vi "read_plc_datasocket.vi"() -> ()   [LabVIEW 2011]
panel:
  out "LB201_B226_GT402":string
  out "LB201_B226_GP102":string
  out "LB201_B226_GT401":string
  out "LB201_B226_GP101":string
  out "LB201_B226_GT301":string
  out "LB201_B226_U201":string
  out "LB201_B226_GT101":string
  out "KB3_B226_U201":string
  out "KB3_B226_GT401":string
  out "KB3_B226_GP101":string
  out "KB3_B226_GT101":string
  out "VS201_B226_GT301":string
  out "VS201_B226_GP101":string
  out "VS201_B226_GT401":string
  out "VS201_B226_GT101":string
  out "VS201_B226_U201":string
  out "Elapsed Time":dbl
  out "Command":string
  out "Up Time":string
  out "Startup Time":string
  out "Version":string
  out "LB201_B230_SV201":string
  out "LB201_B230_SV401":string
  out "LB201_B230_ST902":string
  out "LB201_B230_ST901":string
  out "LB201_A213_SV201":string
  out "LB201_A213_ST902":string
  out "LB201_A235_SV401":string
  out "LB201_A235_SV201":string
  out "LB201_A235_ST902":string
  out "LB201_A235_ST901":string
  out "LB201_A225_SV401":string
  out "LB201_A225_SV201":string
  out "LB201_A225_ST902":string
  out "LB201_A225_ST901":string
  out "LB201_A213_SV401":string
  out "LB201_A213_ST901":string
  out "LB201_B230_GQ101":string
  out "LB201_B230_GT101":string
  out "LB201_A235_GQ101":string
  out "LB201_A235_GT101":string
  out "LB201_B230_GN501":string
  out "LB201_A235_GN501":string
  out "LB201_A225_GT101":string
  out "LB201_A225_GQ101":string
  out "LB201_A225_GN501":string
  out "LB201_A213_GT101":string
  out "LB201_A213_GQ101":string
  out "LB201_A213_GN501":string
  out "Deque error":errorcluster
  out "DataSocket error":errorcluster
  out "# Sent Data":u64
  # "OPC Server Status"
  # "AI PLCs (Per Room)"
  # "AI PLCs (Common)"
  # "AO PLCs (Per Room)"
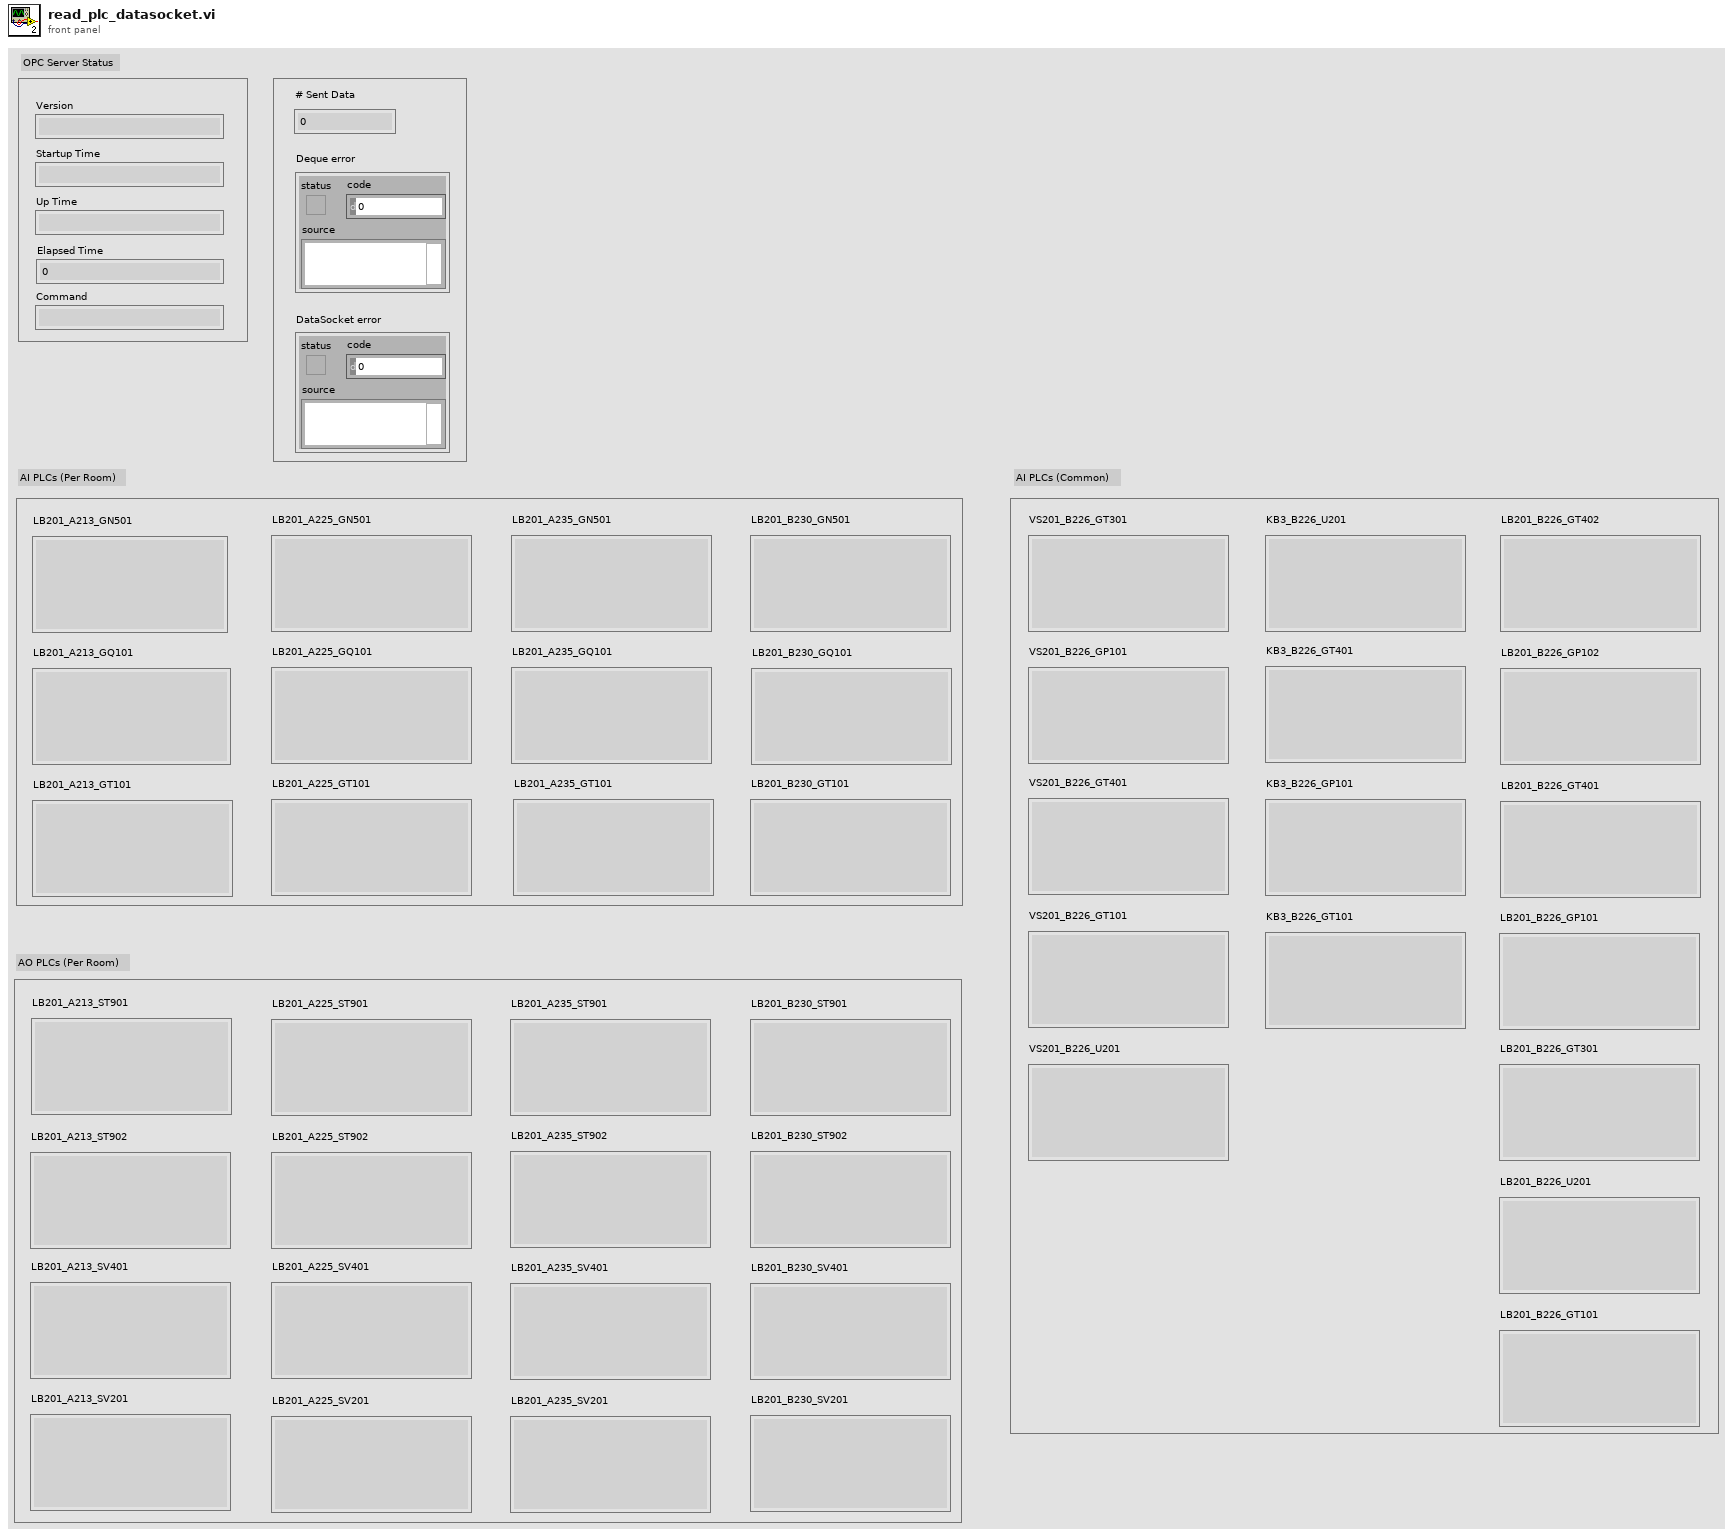
[diagram p1: front panel]
types:
  T1 = enum16{"Read", "Write", "ReadWrite", "BufferedRead", "BufferedReadWrite"}
diagram:
  w3 = string[] ["opc://localhost/Fidelix.FdxOPC/AS_KTH.AI.VS201_B226_GT301_MV.Value", "opc://localhost/Fidelix.FdxOPC/AS_KTH.AI.VS201_B226_GP101_MV.Value", "opc://localhost/Fidelix.FdxOPC/AS_KTH.AI.VS201_B226_GT401_MV.Value", "opc://localhost/Fidelix.FdxOPC/AS_KTH.AI.VS201_B226_GT101_MV.Value", "opc://localhost/Fidelix.FdxOPC/AS_KTH.AI.VS201_B226_U201_SS.Value", "opc://localhost/Fidelix.FdxOPC/AS_KTH.AI.KB3_B226_U201_SS.Value", "opc://localhost/Fidelix.FdxOPC/AS_KTH.AI.KB3_B226_GT401_MV.Value", "opc://localhost/Fidelix.FdxOPC/AS_KTH.AI.KB3_B226_GP101_MV.Value", "opc://localhost/Fidelix.FdxOPC/AS_KTH.AI.KB3_B226_GT101_MV.Value", "opc://localhost/Fidelix.FdxOPC/AS_KTH.AI.LB201_B226_GT402_MV.Value", "opc://localhost/Fidelix.FdxOPC/AS_KTH.AI.LB201_B226_GP102_MV.Value", "opc://localhost/Fidelix.FdxOPC/AS_KTH.AI.LB201_B226_GT401_MV.Value", "opc://localhost/Fidelix.FdxOPC/AS_KTH.AI.LB201_B226_GP101_MV.Value", "opc://localhost/Fidelix.FdxOPC/AS_KTH.AI.LB201_B226_GT301_MV.Value", "opc://localhost/Fidelix.FdxOPC/AS_KTH.AI.LB201_B226_U201_SS.Value", "opc://localhost/Fidelix.FdxOPC/AS_KTH.AI.LB201_B226_GT101_MV.Value"]  # Predefined items
  w32 = string[] ["opc://localhost/Fidelix.FdxOPC/AS_KTH.AI.LB201_A213_ST901_SS.Value", "opc://localhost/Fidelix.FdxOPC/AS_KTH.AI.LB201_A213_ST902_SS.Value", "opc://localhost/Fidelix.FdxOPC/AS_KTH.AI.LB201_A213_SV201_SS.Value", "opc://localhost/Fidelix.FdxOPC/AS_KTH.AI.LB201_A213_SV401_SS.Value", "opc://localhost/Fidelix.FdxOPC/AS_KTH.AI.LB201_A225_ST901_SS.Value", "opc://localhost/Fidelix.FdxOPC/AS_KTH.AI.LB201_A225_ST902_SS.Value", "opc://localhost/Fidelix.FdxOPC/AS_KTH.AI.LB201_A225_SV201_SS.Value", "opc://localhost/Fidelix.FdxOPC/AS_KTH.AI.LB201_A225_SV401_SS.Value", "opc://localhost/Fidelix.FdxOPC/AS_KTH.AI.LB201_A235_ST901_SS.Value", "opc://localhost/Fidelix.FdxOPC/AS_KTH.AI.LB201_A235_ST902_SS.Value", "opc://localhost/Fidelix.FdxOPC/AS_KTH.AI.LB201_A235_SV201_SS.Value", "opc://localhost/Fidelix.FdxOPC/AS_KTH.AI.LB201_A235_SV401_SS.Value", "opc://localhost/Fidelix.FdxOPC/AS_KTH.AI.LB201_B230_ST901_SS.Value", "opc://localhost/Fidelix.FdxOPC/AS_KTH.AI.LB201_B230_ST902_SS.Value", "opc://localhost/Fidelix.FdxOPC/AS_KTH.AI.LB201_B230_SV201_SS.Value", "opc://localhost/Fidelix.FdxOPC/AS_KTH.AI.LB201_B230_SV401_SS.Value"]  # Predefined items
  w37 = string[] ["opc://localhost/Fidelix.FdxOPC/AS_KTH.AI.LB201_A213_GN501_I.Value", "opc://localhost/Fidelix.FdxOPC/AS_KTH.AI.LB201_A213_GQ101_MV.Value", "opc://localhost/Fidelix.FdxOPC/AS_KTH.AI.LB201_A213_GT101_MV.Value", "opc://localhost/Fidelix.FdxOPC/AS_KTH.AI.LB201_A225_GN501_I.Value", "opc://localhost/Fidelix.FdxOPC/AS_KTH.AI.LB201_A225_GQ101_MV.Value", "opc://localhost/Fidelix.FdxOPC/AS_KTH.AI.LB201_A225_GT101_MV.Value", "opc://localhost/Fidelix.FdxOPC/AS_KTH.AI.LB201_A235_GN501_I.Value", "opc://localhost/Fidelix.FdxOPC/AS_KTH.AI.LB201_A235_GQ101_MV.Value", "opc://localhost/Fidelix.FdxOPC/AS_KTH.AI.LB201_A235_GT101_MV.Value", "opc://localhost/Fidelix.FdxOPC/AS_KTH.AI.LB201_B230_GN501_I.Value", "opc://localhost/Fidelix.FdxOPC/AS_KTH.AI.LB201_B230_GQ101_MV.Value", "opc://localhost/Fidelix.FdxOPC/AS_KTH.AI.LB201_B230_GT101_MV.Value"]  # Predefined items
  n1 = for {
    tunnel: w37 -> [w48] mode=indexing
    tunnel: [w47] -> w36 mode=indexing
    tunnel: [w46] -> w35 mode=indexing
    n2 = DataSocket Open(10:T1."Read" ("mode"), 11:w48) -> (0:w46:errorcluster, 3:w47:refnum<k13>)  [unwired: 1 in, 1 out]
  }
  n3 = DataSocket Open(10:T1."Read" ("mode"), 11:"opc://localhost/Fidelix.FdxOPC/ServerStatus.Version" ("URL")) -> (0:w16:errorcluster, 3:w17:refnum<k13>)  [unwired: 1 in, 1 out]
  n4 = DataSocket Open(10:T1."Read" ("mode"), 11:"opc://localhost/Fidelix.FdxOPC/ServerStatus.StartupTime" ("URL")) -> (0:w14:errorcluster, 3:w15:refnum<k13>)  [unwired: 1 in, 1 out]
  n5 = DataSocket Open(10:T1."Read" ("mode"), 11:"opc://localhost/Fidelix.FdxOPC/ServerStatus.UpTime" ("URL")) -> (0:w12:errorcluster, 3:w13:refnum<k13>)  [unwired: 1 in, 1 out]
  n6 = DataSocket Open(10:T1."Read" ("mode"), 11:"opc://localhost/Fidelix.FdxOPC/ServerStatus.ElapsedTime" ("URL")) -> (0:w10:errorcluster, 3:w11:refnum<k13>)  [unwired: 1 in, 1 out]
  n7 = DataSocket Open(10:T1."Read" ("mode"), 11:"opc://localhost/Fidelix.FdxOPC/ServerStatus.Command" ("URL")) -> (0:w8:errorcluster, 3:w9:refnum<k13>)  [unwired: 1 in, 1 out]
  n8 = while {
    tunnel: w17 -> [w58]
    tunnel: w16 -> [w57]
    tunnel: w15 -> [w56]
    tunnel: w14 -> [w55]
    tunnel: w13 -> [w54]
    tunnel: w12 -> [w53]
    tunnel: w11 -> [w52]
    tunnel: w10 -> [w51]
    tunnel: w9 -> [w50]
    tunnel: w8 -> [w49]
    stop <- TRUE continue-if-true
    n9 = DataSocket Read(8:w57, 9:100 ("ms timeout (10000)"), 10:"", 11:w58) -> (2:→"Version":string)  [unwired: 7 out]
    n10 = DataSocket Read(8:w55, 9:100 ("ms timeout (10000)"), 10:"", 11:w56) -> (2:→"Startup Time":string)  [unwired: 7 out]
    n11 = DataSocket Read(8:w53, 9:100 ("ms timeout (10000)"), 10:"", 11:w54) -> (2:→"Up Time":string)  [unwired: 7 out]
    n12 = DataSocket Read(8:w51, 9:100 ("ms timeout (10000)"), 10:0.0, 11:w52) -> (2:→"Elapsed Time":dbl)  [unwired: 7 out]
    n13 = DataSocket Read(8:w49, 9:100 ("ms timeout (10000)"), 10:"", 11:w50) -> (2:→"Command":string)  [unwired: 7 out]
    n14 = Wait Until Next ms Multiple(millisecond multiple=u32 1000) -> ()  [unwired: 1 out]
  }
  n15 = Obtain Queue(max queue size (-1, unlimited)=-1, name (unnamed)="SendingQuePLC", element data type="") -> (queue out=w2:refnum<queue>, error out=w1:errorcluster)  [unwired: 2 in, 1 out]
  n16 = while {
    tunnel: w1 -> [w286]
    tunnel: w2 -> [w285]
    tunnel: w36 -> [w129]
    tunnel: w35 -> [w128]
    tunnel: [w126] -> w34
    tunnel: [w125] -> w33
    stop <- TRUE continue-if-true
    n17 = for {
      tunnel: w129 -> [w292] mode=indexing
      tunnel: [w294] -> w126 mode=indexing
      tunnel: w128 -> [w291] mode=indexing
      tunnel: [w289] -> w127 mode=indexing
      tunnel: [w293] -> w125 mode=indexing
      n18 = DataSocket Read(8:w291, 9:500 ("ms timeout (10000)"), 10:0.0, 11:w292) -> (0:w293:errorcluster, 2:w289:dbl, 3:w294:refnum<k13>)  [unwired: 5 out]
    }
    n19 = Build Array(w127) -> (w76:dbl[][])
    n20 = Index Array(array=w76, index (row)=0, index (col)=0 ("disabled index (col)")) -> (element=w116:dbl)
    n21 = Index Array(array=w76, index (row)=0, index (col)=1 ("disabled index (col)")) -> (element=w99:dbl)
    n22 = Index Array(array=w76, index (row)=0, index (col)=2 ("disabled index (col)")) -> (element=w98:dbl)
    n23 = Index Array(array=w76, index (row)=0, index (col)=3 ("disabled index (col)")) -> (element=w97:dbl)
    n24 = Index Array(array=w76, index (row)=0, index (col)=4 ("disabled index (col)")) -> (element=w96:dbl)
    n25 = Index Array(array=w76, index (row)=0, index (col)=5 ("disabled index (col)")) -> (element=w95:dbl)
    n26 = Index Array(array=w76, index (row)=0, index (col)=6 ("disabled index (col)")) -> (element=w94:dbl)
    n27 = Index Array(array=w76, index (row)=0, index (col)=7 ("disabled index (col)")) -> (element=w93:dbl)
    n28 = Index Array(array=w76, index (row)=0, index (col)=8 ("disabled index (col)")) -> (element=w92:dbl)
    n29 = Index Array(array=w76, index (row)=0, index (col)=9 ("disabled index (col)")) -> (element=w91:dbl)
    n30 = Index Array(array=w76, index (row)=0, index (col)=10 ("disabled index (col)")) -> (element=w90:dbl)
    n31 = Index Array(array=w76, index (row)=0, index (col)=11 ("disabled index (col)")) -> (element=w89:dbl)
    n32 = Wait Until Next ms Multiple(millisecond multiple=u32 30000) -> ()  [unwired: 1 out]
    n33 = Number To Fractional String(number=w98, precision (6)=i16 2) -> (F-format string=w257:string)  [unwired: 2 in]
    n34 = Number To Fractional String(number=w99, precision (6)=i16 2) -> (F-format string=w266:string)  [unwired: 2 in]
    n35 = Number To Fractional String(number=w116, precision (6)=i16 2) -> (F-format string=w279:string)  [unwired: 2 in]
    n36 = Number To Fractional String(number=w95, precision (6)=i16 2) -> (F-format string=w220:string)  [unwired: 2 in]
    n37 = Number To Fractional String(number=w96, precision (6)=i16 2) -> (F-format string=w229:string)  [unwired: 2 in]
    n38 = Number To Fractional String(number=w97, precision (6)=i16 2) -> (F-format string=w242:string)  [unwired: 2 in]
    n39 = Number To Fractional String(number=w94, precision (6)=i16 2) -> (F-format string=w207:string)  [unwired: 2 in]
    n40 = Number To Fractional String(number=w92, precision (6)=i16 2) -> (F-format string=w185:string)  [unwired: 2 in]
    n41 = Number To Fractional String(number=w93, precision (6)=i16 2) -> (F-format string=w176:string)  [unwired: 2 in]
    n42 = Number To Fractional String(number=w91, precision (6)=i16 2) -> (F-format string=w198:string)  [unwired: 2 in]
    n43 = Number To Fractional String(number=w89, precision (6)=i16 2) -> (F-format string=w154:string)  [unwired: 2 in]
    n44 = Number To Fractional String(number=w90, precision (6)=i16 2) -> (F-format string=w163:string)  [unwired: 2 in]
    n45 = Format Date/Time String(time format string (%c)="%y%m%d%H%M%S") -> (date/time string=w256:string)  [unwired: 2 in]
    n46 = Format Date/Time String(time format string (%c)="%y%m%d%H%M%S") -> (date/time string=w267:string)  [unwired: 2 in]
    n47 = Format Date/Time String(time format string (%c)="%y%m%d%H%M%S") -> (date/time string=w278:string)  [unwired: 2 in]
    n48 = Format Date/Time String(time format string (%c)="%y%m%d%H%M%S") -> (date/time string=w219:string)  [unwired: 2 in]
    n49 = Format Date/Time String(time format string (%c)="%y%m%d%H%M%S") -> (date/time string=w230:string)  [unwired: 2 in]
    n50 = Format Date/Time String(time format string (%c)="%y%m%d%H%M%S") -> (date/time string=w241:string)  [unwired: 2 in]
    n51 = Format Date/Time String(time format string (%c)="%y%m%d%H%M%S") -> (date/time string=w208:string)  [unwired: 2 in]
    n52 = Format Date/Time String(time format string (%c)="%y%m%d%H%M%S") -> (date/time string=w186:string)  [unwired: 2 in]
    n53 = Format Date/Time String(time format string (%c)="%y%m%d%H%M%S") -> (date/time string=w175:string)  [unwired: 2 in]
    n54 = Format Date/Time String(time format string (%c)="%y%m%d%H%M%S") -> (date/time string=w197:string)  [unwired: 2 in]
    n55 = Format Date/Time String(time format string (%c)="%y%m%d%H%M%S") -> (date/time string=w153:string)  [unwired: 2 in]
    n56 = Format Date/Time String(time format string (%c)="%y%m%d%H%M%S") -> (date/time string=w164:string)  [unwired: 2 in]
    n57 = Concatenate Strings("GT101" ("string"), "\r", "T" ("string"), "\r", w257, "\r", w256, "\r", "LB201_A213") -> (w260:string)
    "LB201_A213_GT101" <- w260
    n58 = Concatenate Strings("GQ101" ("string"), "\r", "C" ("string"), "\r", w266, "\r", w267, "\r", "LB201_A213") -> (w263:string)
    "LB201_A213_GQ101" <- w263
    n59 = Concatenate Strings("GN501" ("string"), "\r", "M" ("string"), "\r", w279, "\r", w278, "\r", "LB201_A213") -> (w284:string)
    "LB201_A213_GN501" <- w284
    n60 = Concatenate Strings("GT101" ("string"), "\r", "T" ("string"), "\r", w220, "\r", w219, "\r", "LB201_A225") -> (w223:string)
    "LB201_A225_GT101" <- w223
    n61 = Concatenate Strings("GQ101" ("string"), "\r", "C" ("string"), "\r", w229, "\r", w230, "\r", "LB201_A225") -> (w226:string)
    "LB201_A225_GQ101" <- w226
    n62 = Concatenate Strings("GN501" ("string"), "\r", "M" ("string"), "\r", w242, "\r", w241, "\r", "LB201_A225") -> (w245:string)
    "LB201_A225_GN501" <- w245
    n63 = Concatenate Strings("GN501" ("string"), "\r", "M" ("string"), "\r", w207, "\r", w208, "\r", "LB201_A235") -> (w204:string)
    "LB201_A235_GN501" <- w204
    n64 = Concatenate Strings("GT101" ("string"), "\r", "T" ("string"), "\r", w185, "\r", w186, "\r", "LB201_A235") -> (w182:string)
    "LB201_A235_GT101" <- w182
    n65 = Concatenate Strings("GQ101" ("string"), "\r", "C" ("string"), "\r", w176, "\r", w175, "\r", "LB201_A235") -> (w179:string)
    "LB201_A235_GQ101" <- w179
    n66 = Concatenate Strings("GN501" ("string"), "\r", "M" ("string"), "\r", w198, "\r", w197, "\r", "LB201_B230") -> (w201:string)
    "LB201_B230_GN501" <- w201
    n67 = Concatenate Strings("GT101" ("string"), "\r", "T" ("string"), "\r", w154, "\r", w153, "\r", "LB201_B230") -> (w157:string)
    "LB201_B230_GT101" <- w157
    n68 = Concatenate Strings("GQ101" ("string"), "\r", "C" ("string"), "\r", w163, "\r", w164, "\r", "LB201_B230") -> (w160:string)
    "LB201_B230_GQ101" <- w160
    n69 = Enqueue Element(queue=w285, element=w284, error in (no error)=w286) -> (queue out=w250:refnum<queue>, error out=w248:errorcluster)  [unwired: 1 in, 1 out]
    n70 = Enqueue Element(queue=w250, element=w263, error in (no error)=w248) -> (queue out=w249:refnum<queue>, error out=w247:errorcluster)  [unwired: 1 in, 1 out]
    n71 = Enqueue Element(queue=w249, element=w260, error in (no error)=w247) -> (queue out=w147:refnum<queue>, error out=w146:errorcluster)  [unwired: 1 in, 1 out]
    n72 = Enqueue Element(queue=w147, element=w245, error in (no error)=w146) -> (queue out=w145:refnum<queue>, error out=w144:errorcluster)  [unwired: 1 in, 1 out]
    n73 = Enqueue Element(queue=w145, element=w226, error in (no error)=w144) -> (queue out=w143:refnum<queue>, error out=w142:errorcluster)  [unwired: 1 in, 1 out]
    n74 = Enqueue Element(queue=w143, element=w223, error in (no error)=w142) -> (queue out=w141:refnum<queue>, error out=w140:errorcluster)  [unwired: 1 in, 1 out]
    n75 = Enqueue Element(queue=w141, element=w204, error in (no error)=w140) -> (queue out=w139:refnum<queue>, error out=w138:errorcluster)  [unwired: 1 in, 1 out]
    n76 = Enqueue Element(queue=w139, element=w179, error in (no error)=w138) -> (queue out=w137:refnum<queue>, error out=w136:errorcluster)  [unwired: 1 in, 1 out]
    n77 = Enqueue Element(queue=w137, element=w182, error in (no error)=w136) -> (queue out=w135:refnum<queue>, error out=w134:errorcluster)  [unwired: 1 in, 1 out]
    n78 = Enqueue Element(queue=w135, element=w201, error in (no error)=w134) -> (queue out=w133:refnum<queue>, error out=w132:errorcluster)  [unwired: 1 in, 1 out]
    n79 = Enqueue Element(queue=w133, element=w160, error in (no error)=w132) -> (queue out=w131:refnum<queue>, error out=w130:errorcluster)  [unwired: 1 in, 1 out]
    n80 = Enqueue Element(queue=w131, element=w157, error in (no error)=w130) -> ()  [unwired: 1 in, 3 out]
  }
  n81 = for {
    tunnel: w34 -> [w296] mode=indexing
    tunnel: w33 -> [w295] mode=indexing
    n82 = DataSocket Close(8:w295, 11:w296) -> ()  [unwired: 3 out]
  }
  n83 = DataSocket Open(10:T1."Write" ("mode"), 11:"dstp://localhost/plcs" ("URL 3")) -> (0:w39:errorcluster, 3:w40:refnum<k13>)  [unwired: 2 in]
  n84 = while {
    tunnel: w2 -> [w309]
    tunnel: w40 -> [w308]
    tunnel: w39 -> [w303]
    i -> [w301]
    stop <- w302 stop-if-true
    n85 = Dequeue Element(queue=w309) -> (element=w306:string, error out=w305:errorcluster)  [unwired: 2 in, 2 out]
    "Deque error" <- w305
    n86 = To Variant(anything=w306) -> (Variant=w307:variant)
    n87 = DataSocket Write(8:w303, 10:w307, 11:w308) -> (0:w304:errorcluster)  [unwired: 3 out]
    "DataSocket error" <- w304
    n88 = Unbundle By Name(w304) -> ("status"=w298:bool)
    n89 = Unbundle By Name(w305) -> ("status"=w297:bool)
    n90 = Compound Arithmetic op=OR(w298, w297) -> (w302:bool)
    n91 = call "logging.vi"("data"="counter.vi: datasocket error.", "Boolean"=w298) -> ()  [unwired: 1 in]
    n92 = call "logging.vi"("data"="counter.vi: deque error.", "Boolean"=w297) -> ()  [unwired: 1 in]
    "# Sent Data" <- w301
  }
  n93 = for {
    tunnel: w3 -> [w313] mode=indexing
    tunnel: [w312] -> w4 mode=indexing
    tunnel: [w311] -> w5 mode=indexing
    n94 = DataSocket Open(10:T1."Read" ("mode"), 11:w313) -> (0:w311:errorcluster, 3:w312:refnum<k13>)  [unwired: 1 in, 1 out]
  }
  n95 = while {
    tunnel: w4 -> [w580]
    tunnel: w5 -> [w579]
    tunnel: [w577] -> w6
    tunnel: [w576] -> w7
    tunnel: w2 -> [w485]
    tunnel: w1 -> [w484]
    stop <- TRUE continue-if-true
    n96 = for {
      tunnel: w580 -> [w598] mode=indexing
      tunnel: [w600] -> w577 mode=indexing
      tunnel: w579 -> [w597] mode=indexing
      tunnel: [w595] -> w578 mode=indexing
      tunnel: [w599] -> w576 mode=indexing
      n97 = DataSocket Read(8:w597, 9:500 ("ms timeout (10000)"), 10:0.0, 11:w598) -> (0:w599:errorcluster, 2:w595:dbl, 3:w600:refnum<k13>)  [unwired: 5 out]
    }
    n98 = Build Array(w578) -> (w542:dbl[][])
    n99 = Index Array(array=w542, index (row)=0, index (col)=0 ("disabled index (col)")) -> (element=w483:dbl)
    n100 = Index Array(array=w542, index (row)=0, index (col)=1 ("disabled index (col)")) -> (element=w482:dbl)
    n101 = Index Array(array=w542, index (row)=0, index (col)=2 ("disabled index (col)")) -> (element=w481:dbl)
    n102 = Index Array(array=w542, index (row)=0, index (col)=3 ("disabled index (col)")) -> (element=w480:dbl)
    n103 = Index Array(array=w542, index (row)=0, index (col)=4 ("disabled index (col)")) -> (element=w479:dbl)
    n104 = Index Array(array=w542, index (row)=0, index (col)=5 ("disabled index (col)")) -> (element=w422:dbl)
    n105 = Index Array(array=w542, index (row)=0, index (col)=6 ("disabled index (col)")) -> (element=w421:dbl)
    n106 = Index Array(array=w542, index (row)=0, index (col)=7 ("disabled index (col)")) -> (element=w420:dbl)
    n107 = Index Array(array=w542, index (row)=0, index (col)=8 ("disabled index (col)")) -> (element=w419:dbl)
    n108 = Index Array(array=w542, index (row)=0, index (col)=9 ("disabled index (col)")) -> (element=w320:dbl)
    n109 = Index Array(array=w542, index (row)=0, index (col)=10 ("disabled index (col)")) -> (element=w319:dbl)
    n110 = Index Array(array=w542, index (row)=0, index (col)=11 ("disabled index (col)")) -> (element=w318:dbl)
    n111 = Index Array(array=w542, index (row)=0, index (col)=12 ("disabled index (col)")) -> (element=w317:dbl)
    n112 = Index Array(array=w542, index (row)=0, index (col)=13 ("disabled index (col)")) -> (element=w316:dbl)
    n113 = Index Array(array=w542, index (row)=0, index (col)=14 ("disabled index (col)")) -> (element=w315:dbl)
    n114 = Index Array(array=w542, index (row)=0, index (col)=15 ("disabled index (col)")) -> (element=w314:dbl)
    n115 = Wait Until Next ms Multiple(millisecond multiple=u32 30000) -> ()  [unwired: 1 out]
    n116 = Number To Fractional String(number=w482, precision (6)=i16 2) -> (F-format string=w492:string)  [unwired: 2 in]
    n117 = Number To Fractional String(number=w480, precision (6)=i16 2) -> (F-format string=w514:string)  [unwired: 2 in]
    n118 = Number To Fractional String(number=w481, precision (6)=i16 2) -> (F-format string=w505:string)  [unwired: 2 in]
    n119 = Number To Fractional String(number=w483, precision (6)=i16 2) -> (F-format string=w585:string)  [unwired: 2 in]
    n120 = Number To Fractional String(number=w479, precision (6)=i16 2) -> (F-format string=w527:string)  [unwired: 2 in]
    n121 = Number To Fractional String(number=w422, precision (6)=i16 2) -> (F-format string=w474:string)  [unwired: 2 in]
    n122 = Number To Fractional String(number=w420, precision (6)=i16 2) -> (F-format string=w452:string)  [unwired: 2 in]
    n123 = Number To Fractional String(number=w421, precision (6)=i16 2) -> (F-format string=w461:string)  [unwired: 2 in]
    n124 = Number To Fractional String(number=w419, precision (6)=i16 2) -> (F-format string=w439:string)  [unwired: 2 in]
    n125 = Number To Fractional String(number=w319, precision (6)=i16 2) -> (F-format string=w347:string)  [unwired: 2 in]
    n126 = Number To Fractional String(number=w320, precision (6)=i16 2) -> (F-format string=w356:string)  [unwired: 2 in]
    n127 = Number To Fractional String(number=w318, precision (6)=i16 2) -> (F-format string=w334:string)  [unwired: 2 in]
    n128 = Number To Fractional String(number=w317, precision (6)=i16 2) -> (F-format string=w367:string)  [unwired: 2 in]
    n129 = Number To Fractional String(number=w315, precision (6)=i16 2) -> (F-format string=w389:string)  [unwired: 2 in]
    n130 = Number To Fractional String(number=w316, precision (6)=i16 2) -> (F-format string=w380:string)  [unwired: 2 in]
    n131 = Number To Fractional String(number=w314, precision (6)=i16 2) -> (F-format string=w402:string)  [unwired: 2 in]
    n132 = Format Date/Time String(time format string (%c)="%y%m%d%H%M%S") -> (date/time string=w493:string)  [unwired: 2 in]
    n133 = Format Date/Time String(time format string (%c)="%y%m%d%H%M%S") -> (date/time string=w515:string)  [unwired: 2 in]
    n134 = Format Date/Time String(time format string (%c)="%y%m%d%H%M%S") -> (date/time string=w504:string)  [unwired: 2 in]
    n135 = Format Date/Time String(time format string (%c)="%y%m%d%H%M%S") -> (date/time string=w586:string)  [unwired: 2 in]
    n136 = Format Date/Time String(time format string (%c)="%y%m%d%H%M%S") -> (date/time string=w526:string)  [unwired: 2 in]
    n137 = Format Date/Time String(time format string (%c)="%y%m%d%H%M%S") -> (date/time string=w473:string)  [unwired: 2 in]
    n138 = Format Date/Time String(time format string (%c)="%y%m%d%H%M%S") -> (date/time string=w451:string)  [unwired: 2 in]
    n139 = Format Date/Time String(time format string (%c)="%y%m%d%H%M%S") -> (date/time string=w462:string)  [unwired: 2 in]
    n140 = Format Date/Time String(time format string (%c)="%y%m%d%H%M%S") -> (date/time string=w440:string)  [unwired: 2 in]
    n141 = Format Date/Time String(time format string (%c)="%y%m%d%H%M%S") -> (date/time string=w346:string)  [unwired: 2 in]
    n142 = Format Date/Time String(time format string (%c)="%y%m%d%H%M%S") -> (date/time string=w357:string)  [unwired: 2 in]
    n143 = Format Date/Time String(time format string (%c)="%y%m%d%H%M%S") -> (date/time string=w335:string)  [unwired: 2 in]
    n144 = Format Date/Time String(time format string (%c)="%y%m%d%H%M%S") -> (date/time string=w368:string)  [unwired: 2 in]
    n145 = Format Date/Time String(time format string (%c)="%y%m%d%H%M%S") -> (date/time string=w390:string)  [unwired: 2 in]
    n146 = Format Date/Time String(time format string (%c)="%y%m%d%H%M%S") -> (date/time string=w379:string)  [unwired: 2 in]
    n147 = Format Date/Time String(time format string (%c)="%y%m%d%H%M%S") -> (date/time string=w401:string)  [unwired: 2 in]
    n148 = Concatenate Strings("GP101" ("string"), "\r", "P" ("string"), "\r", w492, "\r", w493, "\r", "VS201_B226") -> (w489:string)
    "VS201_B226_GP101" <- w489
    n149 = Concatenate Strings("GT101" ("string"), "\r", "T" ("string"), "\r", w514, "\r", w515, "\r", "VS201_B226") -> (w511:string)
    "VS201_B226_GT101" <- w511
    n150 = Concatenate Strings("GT401" ("string"), "\r", "T" ("string"), "\r", w505, "\r", w504, "\r", "VS201_B226") -> (w508:string)
    "VS201_B226_GT401" <- w508
    n151 = Concatenate Strings("GT301" ("string"), "\r", "T" ("string"), "\r", w585, "\r", w586, "\r", "VS201_B226") -> (w582:string)
    "VS201_B226_GT301" <- w582
    n152 = Concatenate Strings("U201" ("string"), "\r", "V" ("string"), "\r", w527, "\r", w526, "\r", "VS201_B226") -> (w530:string)
    "VS201_B226_U201" <- w530
    n153 = Concatenate Strings("U201" ("string"), "\r", "V" ("string"), "\r", w474, "\r", w473, "\r", "KB3_B226") -> (w477:string)
    "KB3_B226_U201" <- w477
    n154 = Concatenate Strings("GP101" ("string"), "\r", "P" ("string"), "\r", w452, "\r", w451, "\r", "KB3_B226") -> (w455:string)
    "KB3_B226_GP101" <- w455
    n155 = Concatenate Strings("GT401" ("string"), "\r", "T" ("string"), "\r", w461, "\r", w462, "\r", "KB3_B226") -> (w458:string)
    "KB3_B226_GT401" <- w458
    n156 = Concatenate Strings("GT101" ("string"), "\r", "T" ("string"), "\r", w439, "\r", w440, "\r", "KB3_B226") -> (w436:string)
    "KB3_B226_GT101" <- w436
    n157 = Concatenate Strings("GP102" ("string"), "\r", "P" ("string"), "\r", w347, "\r", w346, "\r", "LB201_B226") -> (w350:string)
    "LB201_B226_GP102" <- w350
    n158 = Concatenate Strings("GT402" ("string"), "\r", "T" ("string"), "\r", w356, "\r", w357, "\r", "LB201_B226") -> (w353:string)
    "LB201_B226_GT402" <- w353
    n159 = Concatenate Strings("GT401" ("string"), "\r", "T" ("string"), "\r", w334, "\r", w335, "\r", "LB201_B226") -> (w331:string)
    "LB201_B226_GT401" <- w331
    n160 = Concatenate Strings("GP101" ("string"), "\r", "P" ("string"), "\r", w367, "\r", w368, "\r", "LB201_B226") -> (w364:string)
    "LB201_B226_GP101" <- w364
    n161 = Concatenate Strings("U201" ("string"), "\r", "V" ("string"), "\r", w389, "\r", w390, "\r", "LB201_B226") -> (w386:string)
    "LB201_B226_U201" <- w386
    n162 = Concatenate Strings("GT301" ("string"), "\r", "T" ("string"), "\r", w380, "\r", w379, "\r", "LB201_B226") -> (w383:string)
    "LB201_B226_GT301" <- w383
    n163 = Concatenate Strings("GT101" ("string"), "\r", "T" ("string"), "\r", w402, "\r", w401, "\r", "LB201_B226") -> (w405:string)
    "LB201_B226_GT101" <- w405
    n164 = Enqueue Element(queue=w485, element=w582, error in (no error)=w484) -> (queue out=w486:refnum<queue>, error out=w487:errorcluster)  [unwired: 1 in, 1 out]
    n165 = Enqueue Element(queue=w486, element=w489, error in (no error)=w487) -> (queue out=w532:refnum<queue>, error out=w533:errorcluster)  [unwired: 1 in, 1 out]
    n166 = Enqueue Element(queue=w532, element=w508, error in (no error)=w533) -> (queue out=w534:refnum<queue>, error out=w535:errorcluster)  [unwired: 1 in, 1 out]
    n167 = Enqueue Element(queue=w534, element=w511, error in (no error)=w535) -> (queue out=w536:refnum<queue>, error out=w537:errorcluster)  [unwired: 1 in, 1 out]
    n168 = Enqueue Element(queue=w536, element=w530, error in (no error)=w537) -> (queue out=w424:refnum<queue>, error out=w423:errorcluster)  [unwired: 1 in, 1 out]
    n169 = Enqueue Element(queue=w424, element=w477, error in (no error)=w423) -> (queue out=w434:refnum<queue>, error out=w433:errorcluster)  [unwired: 1 in, 1 out]
    n170 = Enqueue Element(queue=w434, element=w458, error in (no error)=w433) -> (queue out=w432:refnum<queue>, error out=w431:errorcluster)  [unwired: 1 in, 1 out]
    n171 = Enqueue Element(queue=w432, element=w455, error in (no error)=w431) -> (queue out=w430:refnum<queue>, error out=w429:errorcluster)  [unwired: 1 in, 1 out]
    n172 = Enqueue Element(queue=w430, element=w436, error in (no error)=w429) -> (queue out=w321:refnum<queue>, error out=w322:errorcluster)  [unwired: 1 in, 1 out]
    n173 = Enqueue Element(queue=w321, element=w353, error in (no error)=w322) -> (queue out=w329:refnum<queue>, error out=w328:errorcluster)  [unwired: 1 in, 1 out]
    n174 = Enqueue Element(queue=w329, element=w350, error in (no error)=w328) -> (queue out=w327:refnum<queue>, error out=w326:errorcluster)  [unwired: 1 in, 1 out]
    n175 = Enqueue Element(queue=w327, element=w331, error in (no error)=w326) -> (queue out=w417:refnum<queue>, error out=w418:errorcluster)  [unwired: 1 in, 1 out]
    n176 = Enqueue Element(queue=w417, element=w364, error in (no error)=w418) -> (queue out=w407:refnum<queue>, error out=w408:errorcluster)  [unwired: 1 in, 1 out]
    n177 = Enqueue Element(queue=w407, element=w383, error in (no error)=w408) -> (queue out=w409:refnum<queue>, error out=w410:errorcluster)  [unwired: 1 in, 1 out]
    n178 = Enqueue Element(queue=w409, element=w386, error in (no error)=w410) -> (queue out=w411:refnum<queue>, error out=w412:errorcluster)  [unwired: 1 in, 1 out]
    n179 = Enqueue Element(queue=w411, element=w405, error in (no error)=w412) -> ()  [unwired: 1 in, 3 out]
  }
  n180 = for {
    tunnel: w6 -> [w602] mode=indexing
    tunnel: w7 -> [w601] mode=indexing
    n181 = DataSocket Close(8:w601, 11:w602) -> ()  [unwired: 3 out]
  }
  n182 = for {
    tunnel: w32 -> [w606] mode=indexing
    tunnel: [w605] -> w29 mode=indexing
    tunnel: [w604] -> w28 mode=indexing
    n183 = DataSocket Open(10:T1."Read" ("mode"), 11:w606) -> (0:w604:errorcluster, 3:w605:refnum<k13>)  [unwired: 1 in, 1 out]
  }
  n184 = while {
    tunnel: w1 -> [w739]
    tunnel: w2 -> [w677]
    tunnel: [w649] -> w31
    tunnel: [w648] -> w30
    tunnel: w29 -> [w647]
    tunnel: w28 -> [w646]
    stop <- TRUE continue-if-true
    n185 = for {
      tunnel: w647 -> [w876] mode=indexing
      tunnel: [w878] -> w648 mode=indexing
      tunnel: w646 -> [w875] mode=indexing
      tunnel: [w873] -> w676 mode=indexing
      tunnel: [w877] -> w649 mode=indexing
      n186 = DataSocket Read(8:w875, 9:500 ("ms timeout (10000)"), 10:0.0, 11:w876) -> (0:w877:errorcluster, 2:w873:dbl, 3:w878:refnum<k13>)  [unwired: 5 out]
    }
    n187 = Build Array(w676) -> (w639:dbl[][])
    n188 = Index Array(array=w639, index (row)=0, index (col)=15 ("disabled index (col)")) -> (element=w623:dbl)
    n189 = Index Array(array=w639, index (row)=0, index (col)=0 ("disabled index (col)")) -> (element=w638:dbl)
    n190 = Index Array(array=w639, index (row)=0, index (col)=1 ("disabled index (col)")) -> (element=w637:dbl)
    n191 = Index Array(array=w639, index (row)=0, index (col)=2 ("disabled index (col)")) -> (element=w636:dbl)
    n192 = Index Array(array=w639, index (row)=0, index (col)=3 ("disabled index (col)")) -> (element=w635:dbl)
    n193 = Index Array(array=w639, index (row)=0, index (col)=4 ("disabled index (col)")) -> (element=w634:dbl)
    n194 = Index Array(array=w639, index (row)=0, index (col)=5 ("disabled index (col)")) -> (element=w633:dbl)
    n195 = Index Array(array=w639, index (row)=0, index (col)=6 ("disabled index (col)")) -> (element=w632:dbl)
    n196 = Index Array(array=w639, index (row)=0, index (col)=7 ("disabled index (col)")) -> (element=w631:dbl)
    n197 = Index Array(array=w639, index (row)=0, index (col)=8 ("disabled index (col)")) -> (element=w630:dbl)
    n198 = Index Array(array=w639, index (row)=0, index (col)=9 ("disabled index (col)")) -> (element=w629:dbl)
    n199 = Index Array(array=w639, index (row)=0, index (col)=10 ("disabled index (col)")) -> (element=w628:dbl)
    n200 = Index Array(array=w639, index (row)=0, index (col)=11 ("disabled index (col)")) -> (element=w627:dbl)
    n201 = Index Array(array=w639, index (row)=0, index (col)=12 ("disabled index (col)")) -> (element=w626:dbl)
    n202 = Index Array(array=w639, index (row)=0, index (col)=13 ("disabled index (col)")) -> (element=w625:dbl)
    n203 = Index Array(array=w639, index (row)=0, index (col)=14 ("disabled index (col)")) -> (element=w624:dbl)
    n204 = Wait Until Next ms Multiple(millisecond multiple=u32 30000) -> ()  [unwired: 1 out]
    n205 = Number To Fractional String(number=w637, precision (6)=i16 2) -> (F-format string=w855:string)  [unwired: 2 in]
    n206 = Number To Fractional String(number=w638, precision (6)=i16 2) -> (F-format string=w847:string)  [unwired: 2 in]
    n207 = Number To Fractional String(number=w636, precision (6)=i16 2) -> (F-format string=w868:string)  [unwired: 2 in]
    n208 = Number To Fractional String(number=w635, precision (6)=i16 2) -> (F-format string=w834:string)  [unwired: 2 in]
    n209 = Number To Fractional String(number=w634, precision (6)=i16 2) -> (F-format string=w746:string)  [unwired: 2 in]
    n210 = Number To Fractional String(number=w632, precision (6)=i16 2) -> (F-format string=w768:string)  [unwired: 2 in]
    n211 = Number To Fractional String(number=w633, precision (6)=i16 2) -> (F-format string=w759:string)  [unwired: 2 in]
    n212 = Number To Fractional String(number=w631, precision (6)=i16 2) -> (F-format string=w781:string)  [unwired: 2 in]
    n213 = Number To Fractional String(number=w629, precision (6)=i16 2) -> (F-format string=w803:string)  [unwired: 2 in]
    n214 = Number To Fractional String(number=w630, precision (6)=i16 2) -> (F-format string=w812:string)  [unwired: 2 in]
    n215 = Number To Fractional String(number=w628, precision (6)=i16 2) -> (F-format string=w790:string)  [unwired: 2 in]
    n216 = Number To Fractional String(number=w627, precision (6)=i16 2) -> (F-format string=w825:string)  [unwired: 2 in]
    n217 = Number To Fractional String(number=w625, precision (6)=i16 2) -> (F-format string=w710:string)  [unwired: 2 in]
    n218 = Number To Fractional String(number=w626, precision (6)=i16 2) -> (F-format string=w719:string)  [unwired: 2 in]
    n219 = Number To Fractional String(number=w623, precision (6)=i16 2) -> (F-format string=w697:string)  [unwired: 2 in]
    n220 = Number To Fractional String(number=w624, precision (6)=i16 2) -> (F-format string=w689:string)  [unwired: 2 in]
    n221 = Format Date/Time String(time format string (%c)="%y%m%d%H%M%S") -> (date/time string=w856:string)  [unwired: 2 in]
    n222 = Format Date/Time String(time format string (%c)="%y%m%d%H%M%S") -> (date/time string=w846:string)  [unwired: 2 in]
    n223 = Format Date/Time String(time format string (%c)="%y%m%d%H%M%S") -> (date/time string=w867:string)  [unwired: 2 in]
    n224 = Format Date/Time String(time format string (%c)="%y%m%d%H%M%S") -> (date/time string=w835:string)  [unwired: 2 in]
    n225 = Format Date/Time String(time format string (%c)="%y%m%d%H%M%S") -> (date/time string=w747:string)  [unwired: 2 in]
    n226 = Format Date/Time String(time format string (%c)="%y%m%d%H%M%S") -> (date/time string=w769:string)  [unwired: 2 in]
    n227 = Format Date/Time String(time format string (%c)="%y%m%d%H%M%S") -> (date/time string=w758:string)  [unwired: 2 in]
    n228 = Format Date/Time String(time format string (%c)="%y%m%d%H%M%S") -> (date/time string=w780:string)  [unwired: 2 in]
    n229 = Format Date/Time String(time format string (%c)="%y%m%d%H%M%S") -> (date/time string=w802:string)  [unwired: 2 in]
    n230 = Format Date/Time String(time format string (%c)="%y%m%d%H%M%S") -> (date/time string=w813:string)  [unwired: 2 in]
    n231 = Format Date/Time String(time format string (%c)="%y%m%d%H%M%S") -> (date/time string=w791:string)  [unwired: 2 in]
    n232 = Format Date/Time String(time format string (%c)="%y%m%d%H%M%S") -> (date/time string=w824:string)  [unwired: 2 in]
    n233 = Format Date/Time String(time format string (%c)="%y%m%d%H%M%S") -> (date/time string=w709:string)  [unwired: 2 in]
    n234 = Format Date/Time String(time format string (%c)="%y%m%d%H%M%S") -> (date/time string=w720:string)  [unwired: 2 in]
    n235 = Format Date/Time String(time format string (%c)="%y%m%d%H%M%S") -> (date/time string=w698:string)  [unwired: 2 in]
    n236 = Format Date/Time String(time format string (%c)="%y%m%d%H%M%S") -> (date/time string=w688:string)  [unwired: 2 in]
    n237 = Concatenate Strings("ST902" ("string"), "\r", "A" ("string"), "\r", w855, "\r", w856, "\r", "LB201_A213") -> (w731:string)
    "LB201_A213_ST902" <- w731
    n238 = Concatenate Strings("ST901" ("string"), "\r", "A" ("string"), "\r", w847, "\r", w846, "\r", "LB201_A213") -> (w850:string)
    "LB201_A213_ST901" <- w850
    n239 = Concatenate Strings("SV201" ("string"), "\r", "A" ("string"), "\r", w868, "\r", w867, "\r", "LB201_A213") -> (w730:string)
    "LB201_A213_SV201" <- w730
    n240 = Concatenate Strings("SV401" ("string"), "\r", "A" ("string"), "\r", w834, "\r", w835, "\r", "LB201_A213") -> (w831:string)
    "LB201_A213_SV401" <- w831
    n241 = Concatenate Strings("ST901" ("string"), "\r", "A" ("string"), "\r", w746, "\r", w747, "\r", "LB201_A225") -> (w743:string)
    "LB201_A225_ST901" <- w743
    n242 = Concatenate Strings("SV201" ("string"), "\r", "A" ("string"), "\r", w768, "\r", w769, "\r", "LB201_A225") -> (w765:string)
    "LB201_A225_SV201" <- w765
    n243 = Concatenate Strings("ST902" ("string"), "\r", "A" ("string"), "\r", w759, "\r", w758, "\r", "LB201_A225") -> (w762:string)
    "LB201_A225_ST902" <- w762
    n244 = Concatenate Strings("SV401" ("string"), "\r", "A" ("string"), "\r", w781, "\r", w780, "\r", "LB201_A225") -> (w784:string)
    "LB201_A225_SV401" <- w784
    n245 = Concatenate Strings("ST902" ("string"), "\r", "A" ("string"), "\r", w803, "\r", w802, "\r", "LB201_A235") -> (w806:string)
    "LB201_A235_ST902" <- w806
    n246 = Concatenate Strings("ST901" ("string"), "\r", "A" ("string"), "\r", w812, "\r", w813, "\r", "LB201_A235") -> (w809:string)
    "LB201_A235_ST901" <- w809
    n247 = Concatenate Strings("SV201" ("string"), "\r", "A" ("string"), "\r", w790, "\r", w791, "\r", "LB201_A235") -> (w787:string)
    "LB201_A235_SV201" <- w787
    n248 = Concatenate Strings("SV401" ("string"), "\r", "A" ("string"), "\r", w825, "\r", w824, "\r", "LB201_A235") -> (w828:string)
    "LB201_A235_SV401" <- w828
    n249 = Concatenate Strings("ST902" ("string"), "\r", "A" ("string"), "\r", w710, "\r", w709, "\r", "LB201_B230") -> (w713:string)
    "LB201_B230_ST902" <- w713
    n250 = Concatenate Strings("ST901" ("string"), "\r", "A" ("string"), "\r", w719, "\r", w720, "\r", "LB201_B230") -> (w716:string)
    "LB201_B230_ST901" <- w716
    n251 = Concatenate Strings("SV401" ("string"), "\r", "A" ("string"), "\r", w697, "\r", w698, "\r", "LB201_B230") -> (w694:string)
    "LB201_B230_SV401" <- w694
    n252 = Concatenate Strings("SV201" ("string"), "\r", "A" ("string"), "\r", w689, "\r", w688, "\r", "LB201_B230") -> (w680:string)
    "LB201_B230_SV201" <- w680
    n253 = Enqueue Element(queue=w677, element=w850, error in (no error)=w739) -> (error out=w738:errorcluster)  [unwired: 1 in, 2 out]
    n254 = Enqueue Element(queue=w677, element=w731, error in (no error)=w738) -> (error out=w737:errorcluster)  [unwired: 1 in, 2 out]
    n255 = Enqueue Element(queue=w677, element=w730, error in (no error)=w737) -> (error out=w736:errorcluster)  [unwired: 1 in, 2 out]
    n256 = Enqueue Element(queue=w677, element=w831, error in (no error)=w736) -> (error out=w735:errorcluster)  [unwired: 1 in, 2 out]
    n257 = Enqueue Element(queue=w677, element=w743, error in (no error)=w735) -> (error out=w734:errorcluster)  [unwired: 1 in, 2 out]
    n258 = Enqueue Element(queue=w677, element=w762, error in (no error)=w734) -> (error out=w733:errorcluster)  [unwired: 1 in, 2 out]
    n259 = Enqueue Element(queue=w677, element=w765, error in (no error)=w733) -> (error out=w732:errorcluster)  [unwired: 1 in, 2 out]
    n260 = Enqueue Element(queue=w677, element=w784, error in (no error)=w732) -> (error out=w729:errorcluster)  [unwired: 1 in, 2 out]
    n261 = Enqueue Element(queue=w677, element=w809, error in (no error)=w729) -> (error out=w728:errorcluster)  [unwired: 1 in, 2 out]
    n262 = Enqueue Element(queue=w677, element=w806, error in (no error)=w728) -> (error out=w727:errorcluster)  [unwired: 1 in, 2 out]
    n263 = Enqueue Element(queue=w677, element=w787, error in (no error)=w727) -> (error out=w726:errorcluster)  [unwired: 1 in, 2 out]
    n264 = Enqueue Element(queue=w677, element=w828, error in (no error)=w726) -> (error out=w682:errorcluster)  [unwired: 1 in, 2 out]
    n265 = Enqueue Element(queue=w677, element=w716, error in (no error)=w682) -> (error out=w681:errorcluster)  [unwired: 1 in, 2 out]
    n266 = Enqueue Element(queue=w677, element=w713, error in (no error)=w681) -> (error out=w679:errorcluster)  [unwired: 1 in, 2 out]
    n267 = Enqueue Element(queue=w677, element=w680, error in (no error)=w679) -> (error out=w678:errorcluster)  [unwired: 1 in, 2 out]
    n268 = Enqueue Element(queue=w677, element=w694, error in (no error)=w678) -> ()  [unwired: 1 in, 3 out]
  }
  n269 = for {
    tunnel: w30 -> [w880] mode=indexing
    tunnel: w31 -> [w879] mode=indexing
    n270 = DataSocket Close(8:w879, 11:w880) -> ()  [unwired: 3 out]
  }
